vi "Wait.vi"(0 "SecondsWait":u32, 3 "error in":errorcluster) -> (10 "error out":errorcluster)   [LabVIEW 2020]
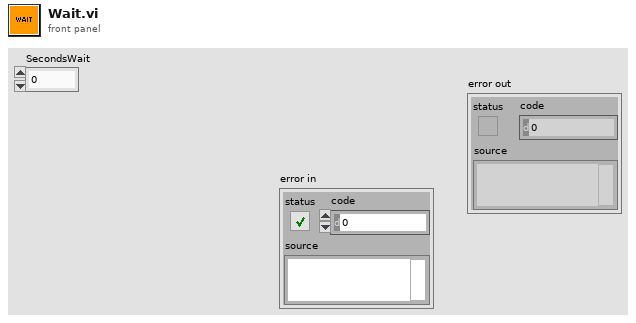
[diagram p1: front panel]
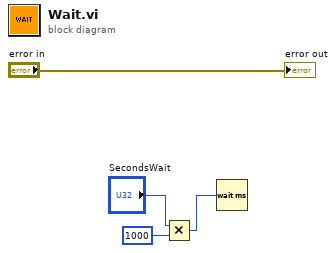
[diagram p0: block diagram]
diagram:
  n1 = Multiply(x="SecondsWait", y=u32 1000) -> (x*y=w1:u32)
  n2 = Wait (ms)(milliseconds to wait=w1) -> ()  [unwired: 1 out]
  "error out" <- "error in"
